vi "Get Properties into Table.vi"(6 "Blacklisted properites":string[](array[string]), 8 "error in":errorcluster, 11 "Item Ref in":T2 format="%.0x") -> (0 "error out":errorcluster, 2 "Property Names":string[][](array[string]), 3 "Item Ref out":T2 format="%.0x")   [LabVIEW 2020, in "AIM ARINC 664 Scripting.lvlib"]
uses:
  AIM ARINC 664 Scripting.lvlib
  <vilib>/NI VeriStand/Custom Device API/Custom Device API.lvlib
  <vilib>/Utility/Data Type/NI_Data Type.lvlib
  <vilib>/NI VeriStand/Custom Device API/Custom Device Item Ref.ctl
  <vilib>/Utility/Data Type/Type Definitions/Data Type.ctl
panel:
  out "type":T1
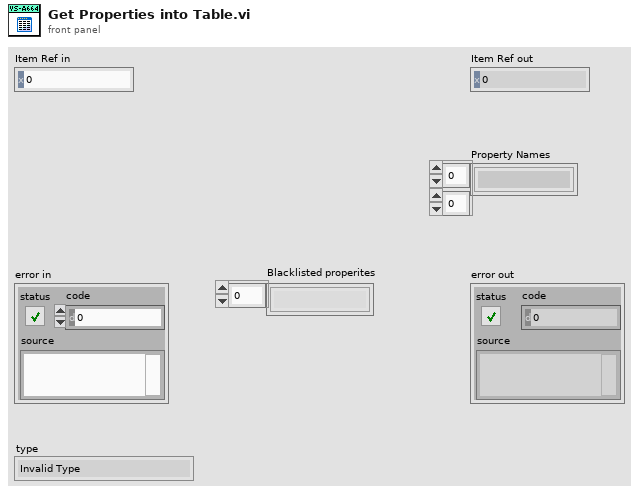
[diagram p1: front panel]
types:
  T1 = typedef "NI_Data Type.lvlib/Data Type.ctl" = enum8{"Invalid Type", "Void", "I8", "I16", "I32", "I64", "U8", "U16", "U32", "U64", "Single Float", "Double Float", "Extended Float", "Single Complex", "Double Complex", "Extended Complex", "Enum U8", "Enum U16", "Enum U32", "Enum U64", "Single Float With Unit", "Double Float With Unit", "Extended Float With Unit", "Single Complex with Unit", "Double Complex with Unit", "Extended Complex with Unit", "Boolean", "String", "Path", "Picture", "Tag", "Array", "Cluster", "Variant", "LV Variant", "Waveform", "Timestamp", "Digital Waveform", "Digital Data", "ExpressData", "Refnum", "External Data", "VI", "Poly VI", "LabVIEW Class Instance", "Fixed Point", "Set Collection", "Map Collection"}
  T2 = typedef "Custom Device API.lvlib/Custom Device Item Ref.ctl" = u64
  T3 = typedef "NI_Data Type.lvlib/Type Definition Info.ctl" = cluster{"Name":string, "Timestamp":u32}
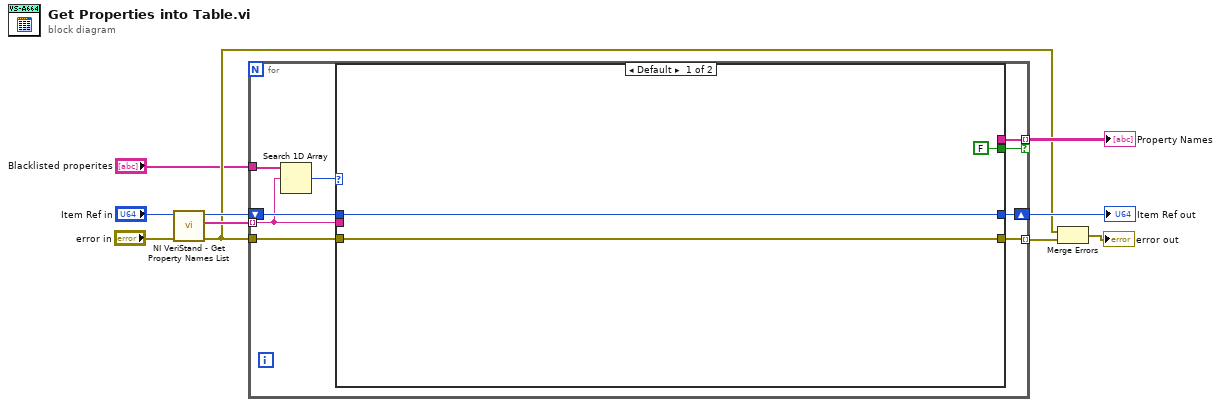
[diagram p0: block diagram]
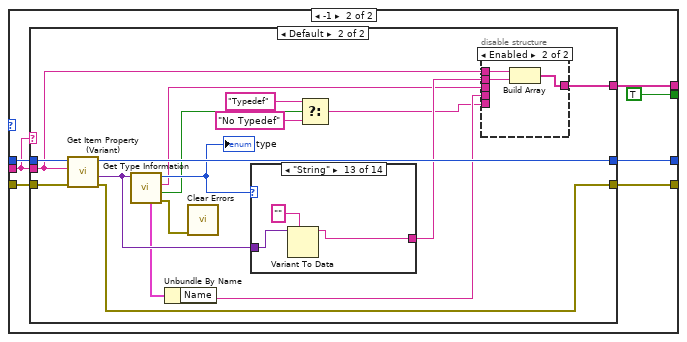
[diagram p2: hidden frame]
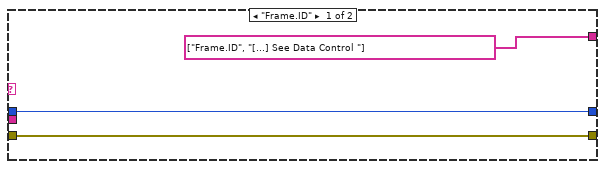
[diagram p3: hidden frame]
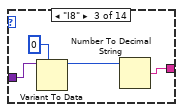
[diagram p6: hidden frame]
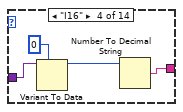
[diagram p7: hidden frame]
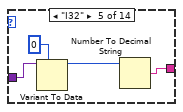
[diagram p8: hidden frame]
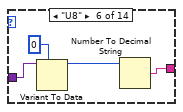
[diagram p9: hidden frame]
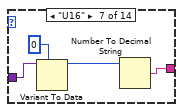
[diagram p10: hidden frame]
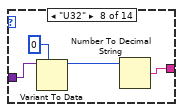
[diagram p11: hidden frame]
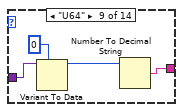
[diagram p12: hidden frame]
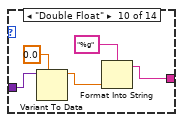
[diagram p13: hidden frame]
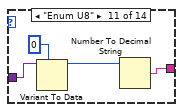
[diagram p14: hidden frame]
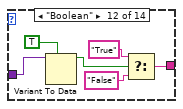
[diagram p15: hidden frame]
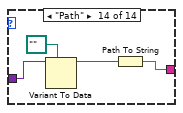
[diagram p16: hidden frame]
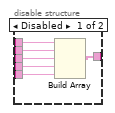
[diagram p17: hidden frame]
diagram:
  n1 = call <vilib>:"NI VeriStand - Get Property Names List.vi"("error in (no error)"="error in", "Item Ref in"="Item Ref in") -> ("error out"=w2:errorcluster, "Property Names"=w8:string[], "Item Ref out"=w7:T2)  [unwired: 7 in]
  n2 = for {
    tunnel: w8 -> [w11] mode=indexing
    shift-right: [w18] -> w6
    shift-left: w7 -> [w19]
    tunnel: w2 -> [w17]
    tunnel: [w16] -> w5 mode=indexing if=w14
    tunnel: [w15] -> w4 mode=indexing
    tunnel: "Blacklisted properites" -> [w13]
    n3 = Search 1D Array(1D array=w13, element=w11) -> (index of element=w12:i32)  [unwired: 1 in]
    n4 = case shown="Default" w12 {
      tunnel: w19 -> [w22 w29]
      tunnel: [w22 w28] -> w18
      tunnel: w17 -> [w21 w27]
      tunnel: [_ w26] -> w16
      tunnel: [w21 w25] -> w15
      tunnel: w11 -> [_ w24]
      tunnel: [FALSE TRUE] -> w14
      frame Default {
      }
      frame -1 {
        n5 = case shown="Default" w24 {
          tunnel: w29 -> [w30 w49]
          tunnel: [w30 w48] -> w28
          tunnel: w27 -> [w31 w47]
          tunnel: w24 -> [_ w44]
          tunnel: [string[] ["Frame.ID", "[...] See Data Control "] w42] -> w26
          tunnel: [w31 w40] -> w25
          frame "Frame.ID" {
          }
          frame Default {
            n6 = call <vilib>:"Get Item Property (Variant).vi"("error in (no error)"=w47, "Property Name"=w44, "Item Ref in"=w49) -> ("error out"=w40:errorcluster, "Value"=w45:variant, "Item Ref out"=w48:T2)  [unwired: 1 in, 5 out]
            n7 = call <vilib>:"Get Type Information.vi"("variant"=w45) -> ("error out"=w41:errorcluster, "type definition"=w36:bool, "name"=w39:string, "type"=w46:T1, "type definition info"=w38:T3)  [unwired: 6 in]
            "type" <- w46
            n8 = Unbundle By Name(w38) -> ("Name"=w37:string)
            n9 = call <vilib>:"Clear Errors.vi"("error in (no error)"=w41) -> ()  [unwired: 5 in, 2 out]
            n10 = case shown="\"String\"" w46 {
              tunnel: w45 -> [_ _ w53 w57 w61 w65 w69 w73 w77 w82 w86 w92 w95 w99]
              tunnel: [_ _ w50 w54 w58 w62 w66 w70 w74 w79 w83 w87 w93 w96] -> w43
              frame "Invalid Type", Default {
              }
              frame "Void" {
              }
              frame "I8" {
                n11 = Variant To Data(type=i8 0, Variant=w53) -> (data=w51:i8)  [unwired: 1 in, 1 out]
                n12 = Number To Decimal String(number=w51) -> (decimal integer string=w50:string)  [unwired: 1 in]
              }
              frame "I16" {
                n13 = Variant To Data(type=i16 0, Variant=w57) -> (data=w55:i16)  [unwired: 1 in, 1 out]
                n14 = Number To Decimal String(number=w55) -> (decimal integer string=w54:string)  [unwired: 1 in]
              }
              frame "I32" {
                n15 = Variant To Data(type=0, Variant=w61) -> (data=w59:i32)  [unwired: 1 in, 1 out]
                n16 = Number To Decimal String(number=w59) -> (decimal integer string=w58:string)  [unwired: 1 in]
              }
              frame "U8" {
                n17 = Variant To Data(type=u8 0, Variant=w65) -> (data=w63:u8)  [unwired: 1 in, 1 out]
                n18 = Number To Decimal String(number=w63) -> (decimal integer string=w62:string)  [unwired: 1 in]
              }
              frame "U16" {
                n19 = Variant To Data(type=u16 0, Variant=w69) -> (data=w67:u16)  [unwired: 1 in, 1 out]
                n20 = Number To Decimal String(number=w67) -> (decimal integer string=w66:string)  [unwired: 1 in]
              }
              frame "U32" {
                n21 = Variant To Data(type=u32 0, Variant=w73) -> (data=w71:u32)  [unwired: 1 in, 1 out]
                n22 = Number To Decimal String(number=w71) -> (decimal integer string=w70:string)  [unwired: 1 in]
              }
              frame "U64" {
                n23 = Variant To Data(type=u64 0, Variant=w77) -> (data=w75:u64)  [unwired: 1 in, 1 out]
                n24 = Number To Decimal String(number=w75) -> (decimal integer string=w74:string)  [unwired: 1 in]
              }
              frame "Double Float" {
                n25 = Variant To Data(type=0.0, Variant=w82) -> (data=w80:dbl)  [unwired: 1 in, 1 out]
                n26 = Format Into String(format string="%g", w80) -> (resulting string=w79:string)  [unwired: 2 in, 1 out]
              }
              frame "Enum U8" {
                n27 = Variant To Data(type=u32 0, Variant=w86) -> (data=w84:u32)  [unwired: 1 in, 1 out]
                n28 = Number To Decimal String(number=w84) -> (decimal integer string=w83:string)  [unwired: 1 in]
              }
              frame "Boolean" {
                n29 = Variant To Data(type=TRUE, Variant=w92) -> (data=w90:bool)  [unwired: 1 in, 1 out]
                n30 = Select(t="True", s=w90, f="False") -> (s? t:f=w87:string)
              }
              frame "String" {
                n31 = Variant To Data(type="", Variant=w95) -> (data=w93:string)  [unwired: 1 in, 1 out]
              }
              frame "Path" {
                n32 = Variant To Data(type=path "", Variant=w99) -> (data=w97:path)  [unwired: 1 in, 1 out]
                n33 = Path To String(path=w97) -> (string=w96:string)
              }
            }
            n34 = Select(t="Typedef" ("Name"), s=w36, f="No Typedef") -> (s? t:f=w33:string)
            n35 = disable-structure shown="Enabled" {
              disable-tunnel: w44 -> [w105 w108]
              disable-tunnel: w43 -> [w104 w107]
              disable-tunnel: [w103 w106] -> w42
              disable-tunnel: w39 -> [w102 _]
              disable-tunnel: w37 -> [w101 _]
              disable-tunnel: w33 -> [w100 _]
              frame Disabled {
                n36 = Build Array(w105, w104, w102, w101, w100) -> (w103:string[])
              }
              frame Enabled {
                n37 = Build Array(w108, w107) -> (w106:string[])
              }
            }
          }
        }
      }
    }
  }
  "Property Names" <- w5
  "Item Ref out" <- w6
  n38 = Merge Errors(w2, w4) -> (→"error out":errorcluster)
